vi "Wiimote Get Acceleration Calibration.vi"(8 "error in":errorcluster, 11 "hWiimoteHandle in":u32 format="%08x") -> (0 "error out":errorcluster, 2 "Calibration Data Out":T2={"Wiimote 0G Calibration"={"Acceleration X"=127.0, "Acceleration Y"=131.0, "Acceleration Z"=126.0}, "Wiimote 1G Calibration"={"Acceleration X"=127.0, "Acceleration Y"=131.0, "Acceleration Z"=126.0}, "Nunchuk 0G Calibration"={"Acceleration X"=127.0, "Acceleration Y"=131.0, "Acceleration Z"=126.0}, "Nunchuk 1G Calibration"={"Acceleration X"=127.0, "Acceleration Y"=131.0, "Acceleration Z"=126.0}}, 3 "hWiimoteHandle out":u32 format="%08x")   [LabVIEW 2011, in "Wiimote.lvlib"]
uses:
  Wiimote.lvlib
  Wiimote Acceleration.ctl
  Wiimote Address Space.ctl
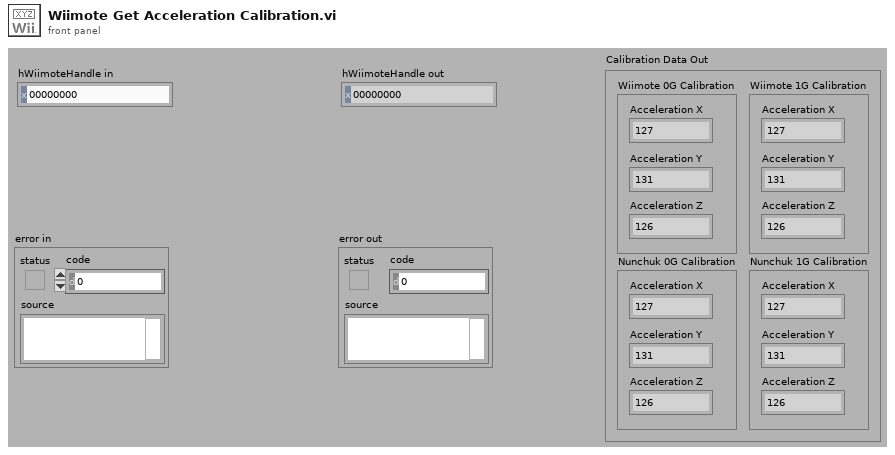
[diagram p1: front panel]
types:
  T1 = typedef "Wiimote.lvlib/Wiimote Acceleration.ctl" = cluster{"Acceleration X":dbl, "Acceleration Y":dbl, "Acceleration Z":dbl}
  T2 = cluster{"Wiimote 0G Calibration":T1, "Wiimote 1G Calibration":T1, "Nunchuk 0G Calibration":T1, "Nunchuk 1G Calibration":T1}
  T3 = typedef "Wiimote.lvlib/Wiimote Address Space.ctl" = u8
  T4 = cluster{cluster{"[0]":dbl, "[1]":dbl, "[2]":dbl}, cluster{"[0]":dbl, "[1]":dbl, "[2]":dbl}, cluster{"[0]":dbl, "[1]":dbl, "[2]":dbl}, cluster{"[0]":dbl, "[1]":dbl, "[2]":dbl}}
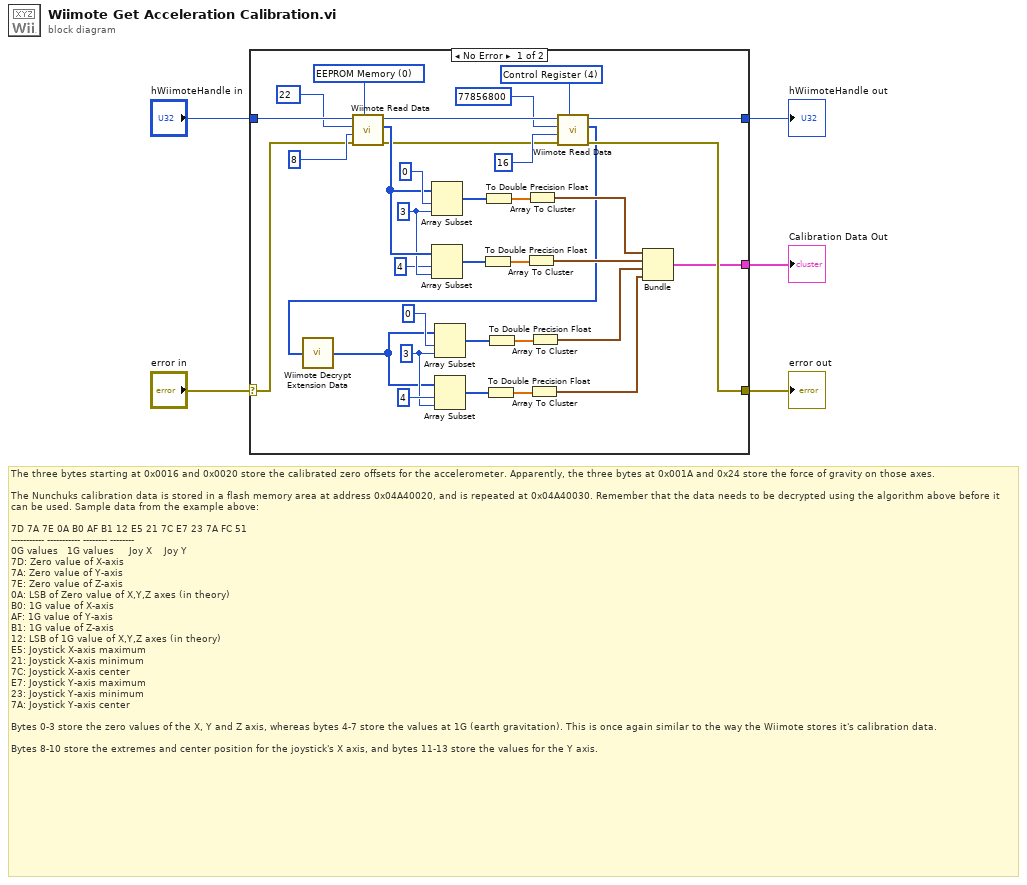
[diagram p0: block diagram]
diagram:
  # "The three bytes starting at 0x0016 and 0x0020 store the calibrated zero offsets for the accelerometer. Apparently, the three bytes at 0x001A and 0x24 store the force of gravity on those axes.\n\nThe Nunchuks calibration data is stored in a flash memory area at address 0x04A40020, and is repeated at 0x04A40030. Remember that the data needs to be decrypted using the algorithm above before it can be used. Sample data from the example above:\n\n7D 7A 7E 0A B0 AF B1 12 E5 21 7C E7 23 7A FC 51\n----------- ----------- -------- --------\n0G values   1G values     Joy X    Joy Y\n7D: Zero value of X-axis\n7A: Zero value of Y-axis\n7E: Zero value of Z-axis\n0A: LSB of Zero value of X,Y,Z axes (in theory)\nB0: 1G value of X-axis\nAF: 1G value of Y-axis\nB1: 1G value of Z-axis\n12: LSB of 1G value of X,Y,Z axes (in theory)\nE5: Joystick X-axis maximum\n21: Joystick X-axis minimum\n7C: Joystick X-axis center\nE7: Joystick Y-axis maximum\n23: Joystick Y-axis minimum\n7A: Joystick Y-axis center\n\nBytes 0-3 store the zero values of the X, Y and Z axis, whereas bytes 4-7 store the values at 1G (earth gravitation). This is once again similar to the way the Wiimote stores it's calibration data.\n\nBytes 8-10 store the extremes and center position for the joystick's X axis, and bytes 11-13 store the values for the Y axis."
  n1 = case shown="No Error" "error in" {
    selector: "error in" -> [w36 w41]
    tunnel: [w20 w41] -> w4
    tunnel: "hWiimoteHandle in" -> [w39 w40]
    tunnel: [w24 w40] -> w2
    tunnel: [w8 _] -> w1
    frame No Error {
      w26 = T3 4 items=["EEPROM Memory"=0, "Control Register"=4] ("Address Space")
      w27 = T3 0 items=["EEPROM Memory"=0, "Control Register"=4] ("Address Space")
      w16 = 3 ("length")
      w31 = 3 ("length")
      n2 = call "Wiimote Read Data.vi"("Address Space"=w27, "error in"=w36, "Size"=u16 8, "Offset"=u32 22, "hWiimoteHandle in"=w39) -> ("error out"=w21:errorcluster, "pReportBuffer out"=w32:u8[], "hWiimoteHandle out"=w25:u32)  [unwired: 4 in]
      n3 = Array Subset(array=w32, index=0, length=w31) -> (w34:u8[])
      n4 = Array Subset(array=w32, index=4, length=w31) -> (w29:u8[])
      n5 = To Double Precision Float(number=w29) -> (double precision float=w28:dbl[])
      n6 = To Double Precision Float(number=w34) -> (double precision float=w33:dbl[])
      n7 = Array To Cluster(array=w28) -> (cluster=w11:cluster{"[0]":dbl, "[1]":dbl, "[2]":dbl})
      n8 = Array To Cluster(array=w33) -> (cluster=w12:cluster{"[0]":dbl, "[1]":dbl, "[2]":dbl})
      n9 = call "Wiimote Read Data.vi"("Address Space"=w26, "error in"=w21, "Size"=u16 16, "Offset"=u32 77856800 ("hWiimoteHandle in"), "hWiimoteHandle in"=w25) -> ("error out"=w20:errorcluster, "pReportBuffer out"=w7:u8[], "hWiimoteHandle out"=w24:u32)  [unwired: 4 in]
      n10 = call "Wiimote Decrypt Extension Data.vi"("Encrypted Data in"=w7) -> ("Decrypted Data out"=w6:u8[])
      n11 = Array Subset(array=w6, index=0, length=w16) -> (w14:u8[])
      n12 = Array Subset(array=w6, index=4, length=w16) -> (w18:u8[])
      n13 = To Double Precision Float(number=w18) -> (double precision float=w19:dbl[])
      n14 = To Double Precision Float(number=w14) -> (double precision float=w15:dbl[])
      n15 = Array To Cluster(array=w19) -> (cluster=w9:cluster{"[0]":dbl, "[1]":dbl, "[2]":dbl})
      n16 = Array To Cluster(array=w15) -> (cluster=w10:cluster{"[0]":dbl, "[1]":dbl, "[2]":dbl})
      n17 = Bundle(w12, w11, w10, w9) -> (w8:T4)  [unwired: 1 in]
    }
    frame Error {
    }
  }
  "error out" <- w4
  "hWiimoteHandle out" <- w2
  "Calibration Data Out" <- w1
